vi "Create Satellite Module.vi"(4 "Manifestation Ancestors":T1, 6 "Kernel LVLib Dir":path=path "D:/Development/Projects/LQ-Bindings/src/LabVIEW/LQ Core", 7 "Template LVLib Path":path=path "D:/Development/Projects/LQ-CodeGen/templates/LabVIEW/Template.lvlib", 8 "Dependency Spec Files":path[](array[path]), 10 "Output Dir":path=path "D:/Development/Projects/LQ-Bindings/src/LabVIEW", 11 "Module Spec. File":path=path "D:/Development/Projects/LQ-CodeGen/data/Qt SVG.json") -> ()   [LabVIEW 2014]
doc: "Copyright (c) 2018 Sze Howe Koh\n\nThis Source Code Form is subject to the terms of the Mozilla Public License, v. 2.0. If a copy of the MPL was not distributed with this file, You can obtain one at http://mozilla.org/MPL/2.0/."
uses:
  Data Structures/Manifestation Ancestors.ctl
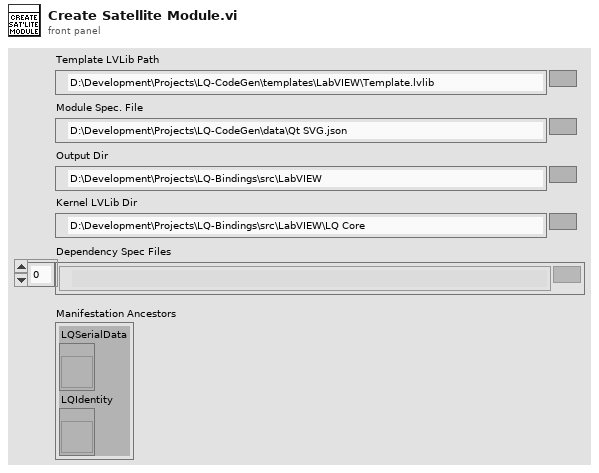
[diagram p1: front panel]
types:
  T1 = typedef "Manifestation Ancestors.ctl" = cluster{"LQSerialData":refnum<vi>, "LQIdentity":refnum<vi>}
  T2 = typedef "Type Categories.ctl" = cluster{"numerics":T3[], "simpleStructs":T4[], "opaqueStructs":T9[], "simpleIdentities":T9[], "qObjects":T9[], "simpleContainers":T3[], "fullArrays":T3[]}
  T3 = typedef "TypeConv.ctl" = cluster{"name":string, "dllType":string}
  T4 = typedef "Simple Struct.ctl" = cluster{"name":string, "fields":T5[], "methods":T6[]}
  T5 = typedef "Param.ctl" = cluster{"name":string, "type":string, "defaultValue":string}
  T6 = typedef "Method.ctl" = cluster{"name":string, "retType":string, "uniqueName":string, "params":T5[], "isConst":bool, "isStaticMember":bool, "isFactory":bool, "connectorPane":T7}
  T7 = typedef "Connector Pane.ctl" = cluster{"pattern":u32, "terminals":T8[]}
  T8 = typedef "Connector Pane Terminal.ctl" = cluster{"name":string, "index":u32}
  T9 = typedef "Class.ctl" = cluster{"name":string, "base":string, "enums":T10[], "methods":T6[], "properties":T12[]}
  T10 = typedef "Enum.ctl" = cluster{"name":string, "values":T11[]}
  T11 = typedef "Enum Value.ctl" = cluster{"name":string, "value":i32}
  T12 = typedef "Property.ctl" = cluster{"name":string, "getter":string, "setter":string}
  T13 = typedef "Namespace.ctl" = cluster{"name":string, "enums":T10[], "methods":T6[]}
  T14 = typedef "Projection Info.ctl" = cluster{"source":string, "projection":string}
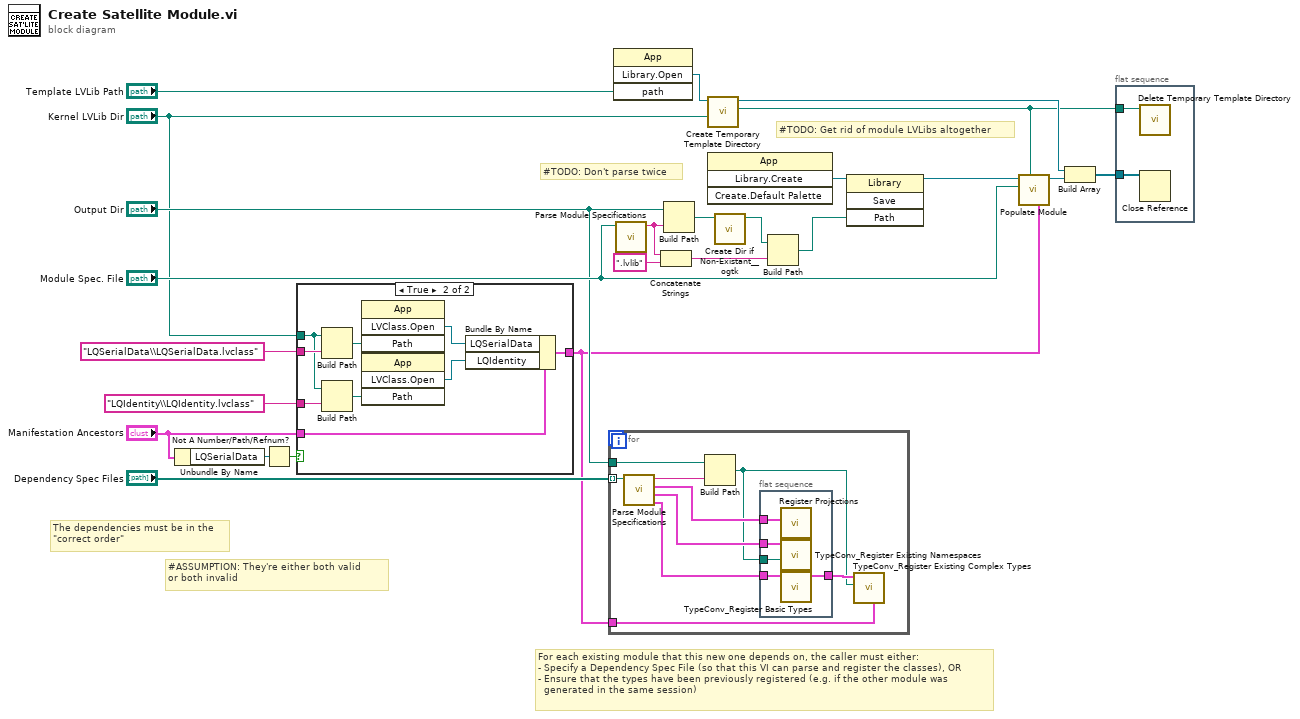
[diagram p0: block diagram]
diagram:
  # "#ASSUMPTION: They're either both valid\nor both invalid"
  # "#TODO: Get rid of module LVLibs altogether"
  # "For each existing module that this new one depends on, the caller must either:\n- Specify a Dependency Spec File (so that this VI can parse and register the classes), OR\n- Ensure that the types have been previously registered (e.g. if the other module was\n  generated in the same session)"
  # "The dependencies must be in the\n\"correct order\""
  # "#TODO: Don't parse twice"
  n1 = Unbundle By Name("Manifestation Ancestors") -> ("LQSerialData"=w4:refnum<vi>)
  n2 = Not A Number/Path/Refnum?(number/path/refnum=w4) -> (NaN/Path/Refnum?=w3:bool)
  n3 = case shown="True" w3 {
    tunnel: "LQSerialData\\LQSerialData.lvclass" ("name or relative path") -> [_ w34]
    tunnel: "LQIdentity\\LQIdentity.lvclass" ("name or relative path") -> [_ w33]
    tunnel: "Kernel LVLib Dir" -> [_ w30]
    tunnel: "Manifestation Ancestors" -> [w25 w29]
    tunnel: [w25 w26] -> w1
    frame False {
    }
    frame True {
      n4 = Build Path(base path=w30, name or relative path=w34) -> (appended path=w32:path)
      n5 = Build Path(base path=w30, name or relative path=w33) -> (appended path=w31:path)
      n6 = invoke class="App" method="LVClass.Open"("Path"=w32) -> ("LVClass.Open"=w28:refnum<vi>)  [unwired: 3 in, 3 out]
      n7 = invoke class="App" method="LVClass.Open"("Path"=w31) -> ("LVClass.Open"=w27:refnum<vi>)  [unwired: 3 in, 3 out]
      n8 = Bundle By Name(cluster=w29, "LQSerialData"=w28, "LQIdentity"=w27) -> (w26:T1)
    }
  }
  n9 = for {
    tunnel: "Dependency Spec Files" -> [w43] mode=indexing
    tunnel: "Output Dir" -> [w41]
    tunnel: w1 -> [w36]
    n10 = call "Parse Module Specifications.vi"("Module Spec. File"=w43) -> ("Type Categories"=w42:T2, "Namespaces"=w38:T13[], "Projections"=w39:T14[], "Module Name"=w40:string)  [unwired: 6 in, 1 out]
    n11 = Build Path(base path=w41, name or relative path=w40) -> (appended path=w35:path)
    n12 = flat-sequence {
      tunnel: w42 -> [w48]
      tunnel: w39 -> [w47]
      tunnel: w38 -> [w46]
      tunnel: [w45] -> w37
      tunnel: w35 -> [w44]
      frame #0 {
        n13 = call "Register Projections.vi"("Projection Info"=w47) -> ()  [unwired: 11 in]
        n14 = call "TypeConv_Register Existing Namespaces.vi"("Existing Module Root Dir"=w44, "Namespaces"=w46) -> ()  [unwired: 10 in]
        n15 = call "TypeConv_Register Basic Types.vi"("Type Categories"=w48) -> ("Type Categories Dup"=w45:T2)  [unwired: 10 in]
      }
    }
    n16 = call "TypeConv_Register Existing Complex Types.vi"("Manifestation Ancestors"=w36, "Module Root Dir"=w35, "Type Categories"=w37) -> ()  [unwired: 8 in, 1 out]
  }
  n17 = invoke class="App" method="Library.Open"("path"="Template LVLib Path") -> ("Open Library"=w21:refnum<vi>)  [unwired: 3 in, 3 out]
  n18 = call "Parse Module Specifications.vi"("Module Spec. File"="Module Spec. File") -> ("Module Name"=w14:string)  [unwired: 6 in, 4 out]
  n19 = Concatenate Strings(w14, ".lvlib" ("string")) -> (w13:string)
  n20 = Build Path(base path="Output Dir", name or relative path=w14) -> (appended path=w17:path)
  n21 = call "Create Temporary Template Directory.vi"("Kernel LVLib Dir"="Kernel LVLib Dir", "Template LVLib"=w21) -> ("Temporary Template Root Dir"=w11:path, "Template LVLib Dup"=w23:refnum<vi>)  [unwired: 8 in]
  n22 = invoke class="App" method="Library.Create"() -> ("Create Library"=w20:refnum<vi>)  [unwired: 4 in, 3 out]
  n23 = call <userlib>:"Create Dir if Non-Existant__ogtk.vi"("Directory Path"=w17) -> ("dup Directory Path"=w16:path)  [unwired: 8 in, 2 out]
  n24 = Build Path(base path=w16, name or relative path=w13) -> (appended path=w12:path)
  n25 = invoke class="Library" method="Save"(reference=w20, "Path"=w12) -> (reference out=w19:refnum<vi>)  [unwired: 2 in, 3 out]
  n26 = call "Populate Module.vi"("Manifestation Ancestors"=w1, "Temporary Template Root Dir"=w11, "Module Spec. File"="Module Spec. File", "Module LVLib"=w19) -> ("Module LVLib Dup"=w9:refnum<vi>)  [unwired: 7 in]
  n27 = Build Array(w23, w9) -> (w24:refnum<vi>[])
  n28 = flat-sequence {
    tunnel: w24 -> [w50]
    tunnel: w11 -> [w49]
    frame #0 {
      n29 = call "Delete Temporary Template Directory.vi"("Target Template Root Dir"=w49) -> ()  [unwired: 11 in]
      n30 = Close Reference(reference=w50) -> ()  [unwired: 1 in, 1 out]
    }
  }
